vi "Login.vi"() -> ()   [LabVIEW 2020]
panel:
  in  "Login":bool
  in  "Cancel":bool
  in  "Password":string
  in  "User Name":string
  # "Smart Home"
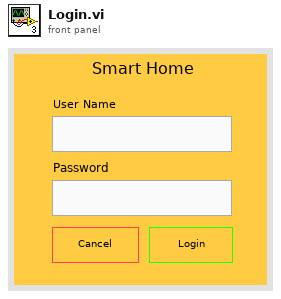
[diagram p1: front panel]
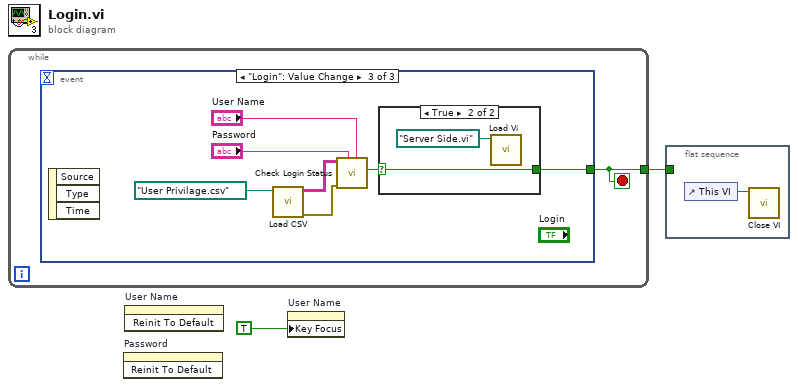
[diagram p0: block diagram]
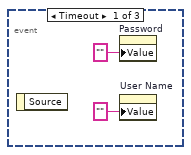
[diagram p2: hidden frame]
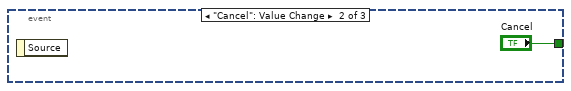
[diagram p3: hidden frame]
diagram:
  n1 = while {
    tunnel: [w3] -> w2
    stop <- w3 stop-if-true
    n2 = event shown="[2] \"Login\": Value Change" {
      selector: _ -> [_ _ _]
      dyn-events: _ -> [_ _ _]
      timeout: _ -> [_ _ _]
      tunnel: [_ "Cancel" w7] -> w3
      event Timeout {
        n3 = event-data() -> ()  [unwired: 1 in, 1 out]
        n4 = property on="Password" class="Str"("Value"="" ("Password")) -> ()  [unwired: 2 in, 2 out]
        n5 = property on="User Name" class="Str"("Value"="" ("User Name")) -> ()  [unwired: 2 in, 2 out]
      }
      event "Cancel": Value Change {
        n6 = event-data() -> ()  [unwired: 1 in, 1 out]
      }
      event "Login": Value Change {
        n7 = event-data() -> ()  [unwired: 1 in, 3 out]
        n8 = call "Load CSV.vi"("File Name"=path "User Privilage.csv" ("name or relative path")) -> ("error out"=w11:errorcluster, "rows"=w12:string[][])  [unwired: 9 in]
        n9 = call "Check Login Status.vi"("User Name"="User Name", "Password"="Password", "error in (no error)"=w11, "rows"=w12) -> ("Status"=w8:bool)  [unwired: 5 in, 2 out]
        n10 = case shown="True" w8 {
          selector: w8 -> [w14 w15]
          tunnel: [w14 w15] -> w7
          frame False {
          }
          frame True {
            n11 = call "Load Vi.vi"("vi path"=path "Server Side.vi") -> ()  [unwired: 10 in, 1 out]
          }
        }
      }
    }
  }
  n12 = invoke on="Password" class="Str" method="Reinit To Default"() -> ()  [unwired: 3 in, 3 out]
  n13 = invoke on="User Name" class="Str" method="Reinit To Default"() -> ()  [unwired: 3 in, 3 out]
  n14 = property on="User Name" class="Str"("Key Focus"=TRUE) -> ()  [unwired: 2 in, 2 out]
  n15 = flat-sequence {
    tunnel: w2 -> [_]
    frame #0 {
      n16 = control-ref of="This VI"() -> (w17:refnum<vi>)
      n17 = call "Close VI.vi"("VI in"=w17) -> ()  [unwired: 11 in]
    }
  }
